vi "Begin.vi"() -> (0 "Error Out":errorcluster)   [LabVIEW 2020]
doc: "This VI opens device references, sets constants, clears hardware sticky faults, defines static VI references, and resets gobal variables."
uses:
  dsdata.vi
  <vilib>/Rock Robotics/WPI/DriverStation/WPI_DriverStationRobotMode2.ctl
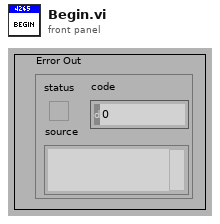
[diagram p1: front panel]
types:
  T1 = typedef "WPI_DriverStationRobotMode2.ctl" = enum16{"Autonomous Disabled", "Autonomous Enabled", "Teleop Disabled", "Teleop Enabled", "Disconnected", "Finish", "Test Disabled", "Test Enabled", "Emergency Stopped"}
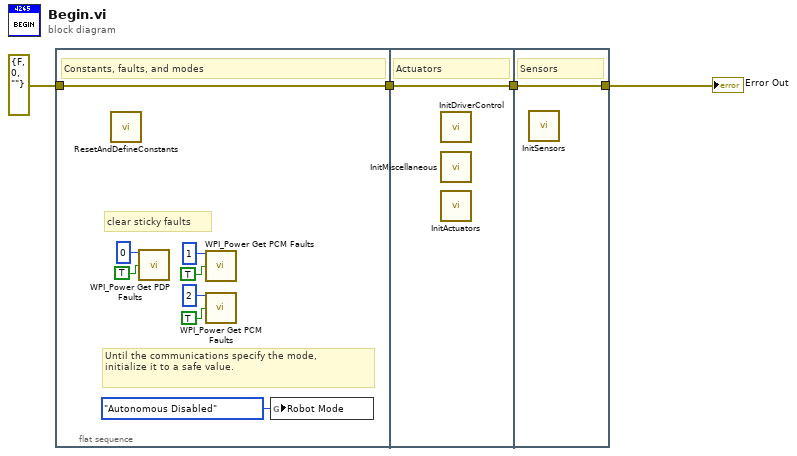
[diagram p0: block diagram]
diagram:
  n1 = flat-sequence {
    tunnel: [w12] -> w4
    tunnel: errorcluster {"status"=FALSE, "code"=0, "source"=""} ("error in") -> [w12]
    tunnel: w4 -> [w13]
    tunnel: [w13] -> w2
    tunnel: w2 -> [w14]
    tunnel: [w14] -> w1
    frame #0 {
      # "clear sticky faults"
      # "Until the communications specify the mode,\ninitialize it to a safe value."
      # "Constants, faults, and modes"
      n2 = call "ResetAndDefineConstants.vi"() -> ()  [unwired: 1 in]
      n3 = call <vilib>:"WPI_Power Get PDP Faults.vi"("Power Distribution (def)"=u8 0 ("Power Distribution Panel (0)"), "Clear Sticky Faults"=TRUE) -> ()  [unwired: 9 in, 5 out]
      n4 = call <vilib>:"WPI_Power Get PCM Faults.vi"("Pneumatics Control Module (0)"=u8 1, "Clear Sticky Faults"=TRUE) -> ()  [unwired: 10 in, 4 out]
      n5 = call <vilib>:"WPI_Power Get PCM Faults.vi"("Pneumatics Control Module (0)"=u8 2, "Clear Sticky Faults"=TRUE) -> ()  [unwired: 10 in, 4 out]
      n6 = global write "dsdata.vi" "Robot Mode"(WPI_DriverStationRobotMode2."Autonomous Disabled" ("Robot Mode")) -> ()
    }
    frame #1 {
      # "Actuators"
      n7 = call "InitDriverControl.vi"() -> ()  [unwired: 12 in]
      n8 = call "InitMiscellaneous.vi"() -> ()  [unwired: 12 in]
      n9 = call "InitActuators.vi"() -> ()  [unwired: 1 in]
    }
    frame #2 {
      # "Sensors"
      n10 = call "InitSensors.vi"() -> ()  [unwired: 1 in]
    }
  }
  "Error Out" <- w1
